vi "WriteConfigKeys.vi"(0 "GRMActor in":refnum<class "GRMActor.lvclass">, 5 "Config Refnum":T1, 7 "Keys":string[](array[string]), 9 "Value":i32[](array[numeric]), 11 "error in (no error)":errorcluster) -> (4 "GRMActor out":refnum<class "GRMActor.lvclass">, 15 "error out":errorcluster)   [LabVIEW 2020, in "GRMActor.lvlib" / "GRMActor.lvclass"]
uses:
  GRMActor.lvclass
  <vilib>/Utility/config.llb/Config Data RefNum.ctl
  <vilib>/Utility/config.llb/Write Key (I32).vi
  <vilib>/Utility/config.llb/NI_LVConfig.lvlib
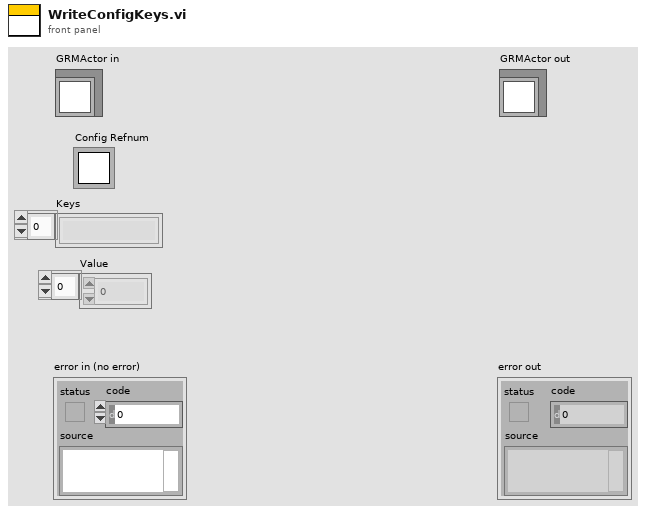
[diagram p1: front panel]
types:
  T1 = typedef "NI_LVConfig.lvlib/Config Data RefNum.ctl" = refnum<k1>
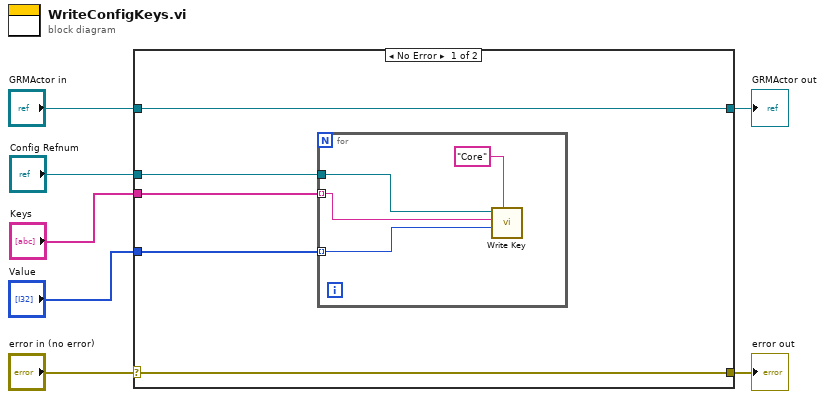
[diagram p0: block diagram]
diagram:
  n1 = case shown="No Error" "error in (no error)" {
    selector: "error in (no error)" -> [w11 w18]
    tunnel: [w11 w18] -> w6
    tunnel: [w12 w17] -> w4
    tunnel: "GRMActor in" -> [w12 w17]
    tunnel: "Config Refnum" -> [w10 _]
    tunnel: "Keys" -> [w9 _]
    tunnel: "Value" -> [w8 _]
    frame No Error {
      n2 = for {
        tunnel: w10 -> [w15]
        tunnel: w9 -> [w14] mode=indexing
        tunnel: w8 -> [w13] mode=indexing
        n3 = call-poly <vilib>:"Write Key.vi"("section"="Core", "value"=w13, "key"=w14, "refnum"=w15) -> ()  [unwired: 5 in, 3 out]
      }
    }
    frame Error {
    }
  }
  "error out" <- w6
  "GRMActor out" <- w4
